vi "Distance Between Line Point.vi"(9 "Point":T2, 11 "Line":T1) -> (3 "Distance":sgl)   [LabVIEW 2020, in "3D Plot.lvclass"]
uses:
  3D Plot.lvclass
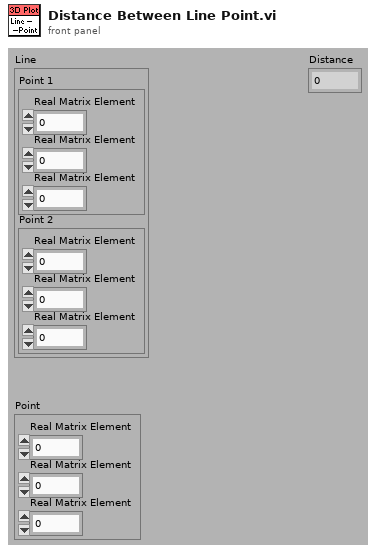
[diagram p1: front panel]
types:
  T1 = cluster{"Point 1":cluster{"Real Matrix Element":sgl, "Real Matrix Element":sgl, "Real Matrix Element":sgl}, "Point 2":cluster{"Real Matrix Element":sgl, "Real Matrix Element":sgl, "Real Matrix Element":sgl}}
  T2 = cluster{"Real Matrix Element":sgl, "Real Matrix Element":sgl, "Real Matrix Element":sgl}
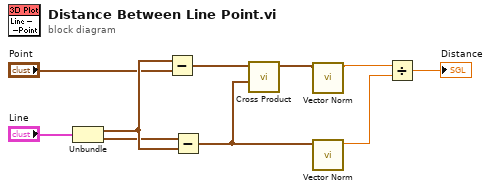
[diagram p0: block diagram]
diagram:
  n1 = Unbundle("Line") -> ("Point 1"=w10:T2, "Point 2"=w9:T2)
  n2 = Subtract(x=w10, y="Point") -> (x-y=w5:T2)
  n3 = Subtract(x=w9, y=w10) -> (x-y=w3:T2)
  n4 = call "Cross Product.vi"("Vector 2"=w3, "Vector 1"=w5) -> ("Vector Out"=w4:cluster{"X":sgl, "Y":sgl, "Z":sgl})  [unwired: 9 out]
  n5 = call "Vector Norm.vi"("Vector"=w4) -> ("Norm"=w1:sgl)  [unwired: 10 out]
  n6 = call "Vector Norm.vi"("Vector"=w3) -> ("Norm"=w2:sgl)  [unwired: 10 out]
  n7 = Divide(x=w1, y=w2) -> (x/y=→"Distance":sgl)
